vi "Error_5112.vi"(11 "Status Byte":i32) -> (0 "error out":errorcluster)   [LabVIEW 2015, in "Tool Module.lvlib"]
uses:
  Tool Module.lvlib
  <vilib>/Utility/error.llb/Error Cluster From Error Code.vi
  <vilib>/ErrorRing/Error Ring.xnode
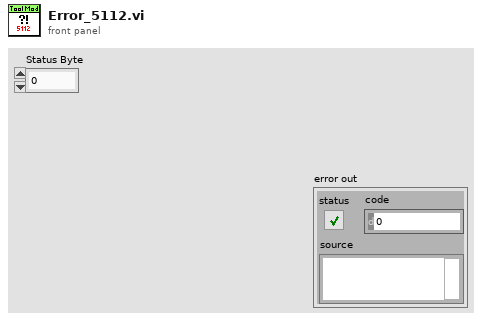
[diagram p1: front panel]
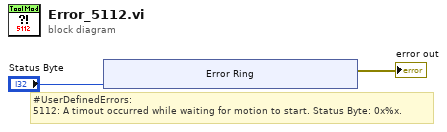
[diagram p0: block diagram]
diagram:
  # "#UserDefinedErrors:\n5112: A timout occurred while waiting for motion to start. Status Byte: 0x%x."
  n1 = xnode "Error Ring"("parameter 0"="Status Byte") -> ("error out"=→"error out":errorcluster)
